vi "2283_mapaLIDAR.vi"(6 "Boolean Shift Register In":bool, 7 "Numeric Shift Register In":i32, 8 "X":dbl=350.0, 9 "# de Lecturas":i32=20) -> (1 "Boolean Shift Register Out":bool, 2 "Num Shift Register Out":i32)   [LabVIEW 2014]
uses:
  Mapa Global.vi
panel:
  out "Polar Plot":picture
  in  "Visible Section":u16(ring)=8
  in  "Grid Color":u32(colorbox)
  in  "Plot Color":u32(colorbox)=16715776
  out "Distance":dbl
  out "Mapa":cluster{dbl[], dbl[]}(graph)
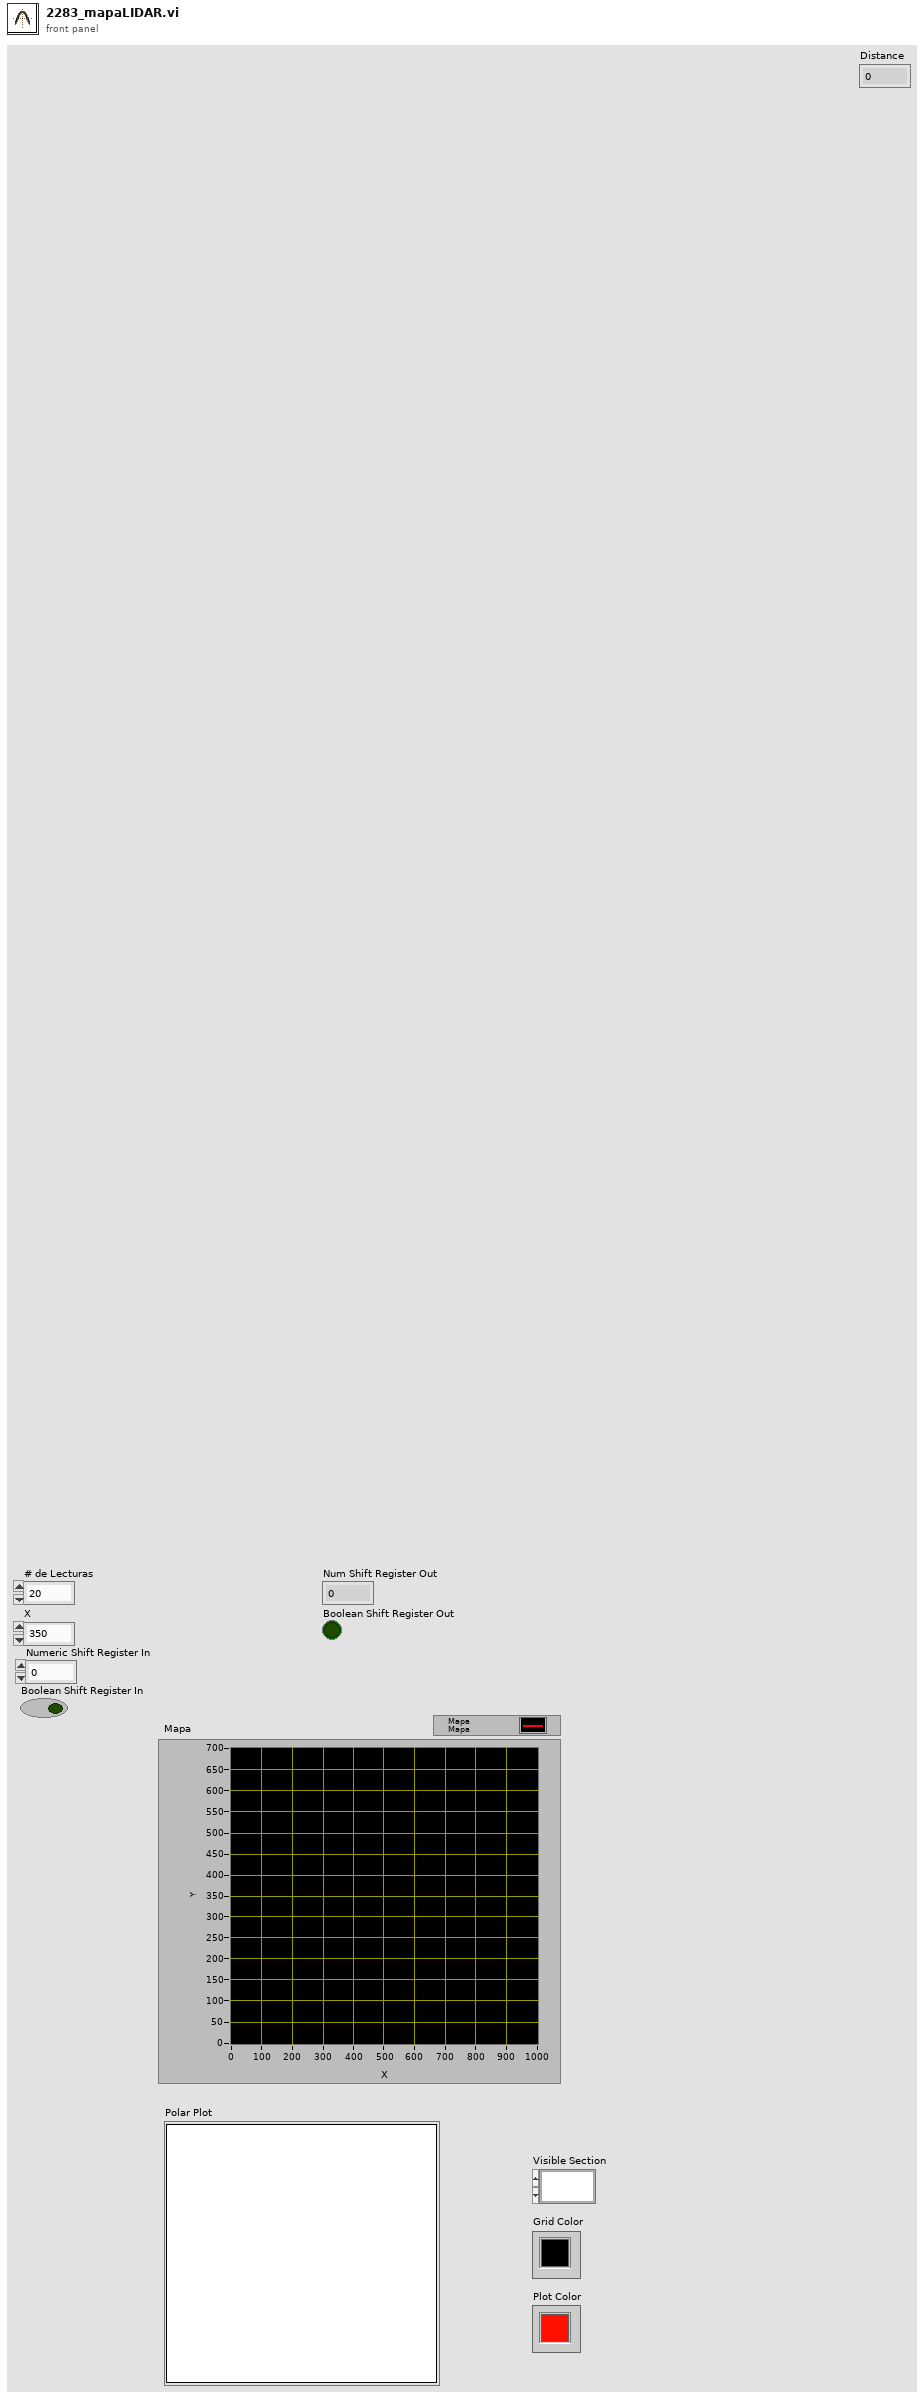
[diagram p1: front panel]
types:
  T1 = cluster{"maximum":dbl, "minimum":dbl, "clip to min":bool, "log?(F)":bool, "grid color":u32, "plot color":u32, "format and precision":cluster{"format":enum8{"Decimal", "Scientific", "Engineering", "Binary", "Octal", "Hex"}, "precision":u8}, "visible section":u16}
  T2 = typedef "WPI_I2CDevRef.ctl" = cluster{"DevStatus":errorcluster, "Controller":T3, "Device Address":u8, "Handle":i32, "I2C Bus":T4}
  T3 = typedef "FPGA_TypedefDigitalModule.ctl" = enum16{"Controller 1"}
  T4 = typedef "i2c_bus.ctl" = enum16{"I2C On-Board", "I2C MXP", "Invalid"}
  T5 = typedef "LVBoundsTypeDef.ctl" = cluster{"Width":u32, "Height":u32}
  T6 = typedef "WPI_ServoDeviceRef.ctl" = cluster{"DeviceStatus":errorcluster, "Controller":T3, "PWM Channel":T7, "DeadBand":T8}
  T7 = typedef "FPGA_DIOPWMChannel.ctl" = enum8{"PWM 0", "PWM 1", "PWM 2", "PWM 3", "PWM 4", "PWM 5", "PWM 6", "PWM 7", "PWM 8", "PWM 9", "PWM MXP 0", "PWM MXP 1", "PWM MXP 2", "PWM MXP 3", "PWM MXP 4", "PWM MXP 5", "PWM MXP 6", "PWM MXP 7", "PWM MXP 8", "PWM MXP 9", "Invalid"}
  T8 = typedef "WPI_PWMDeadband.ctl" = cluster{"Name":string, "maxPositivePwm":i32, "minPositivePwm":i32, "centerPwm":i32, "maxNegativePwm":i32, "minNegativePwm":i32, "angularRange":u16}
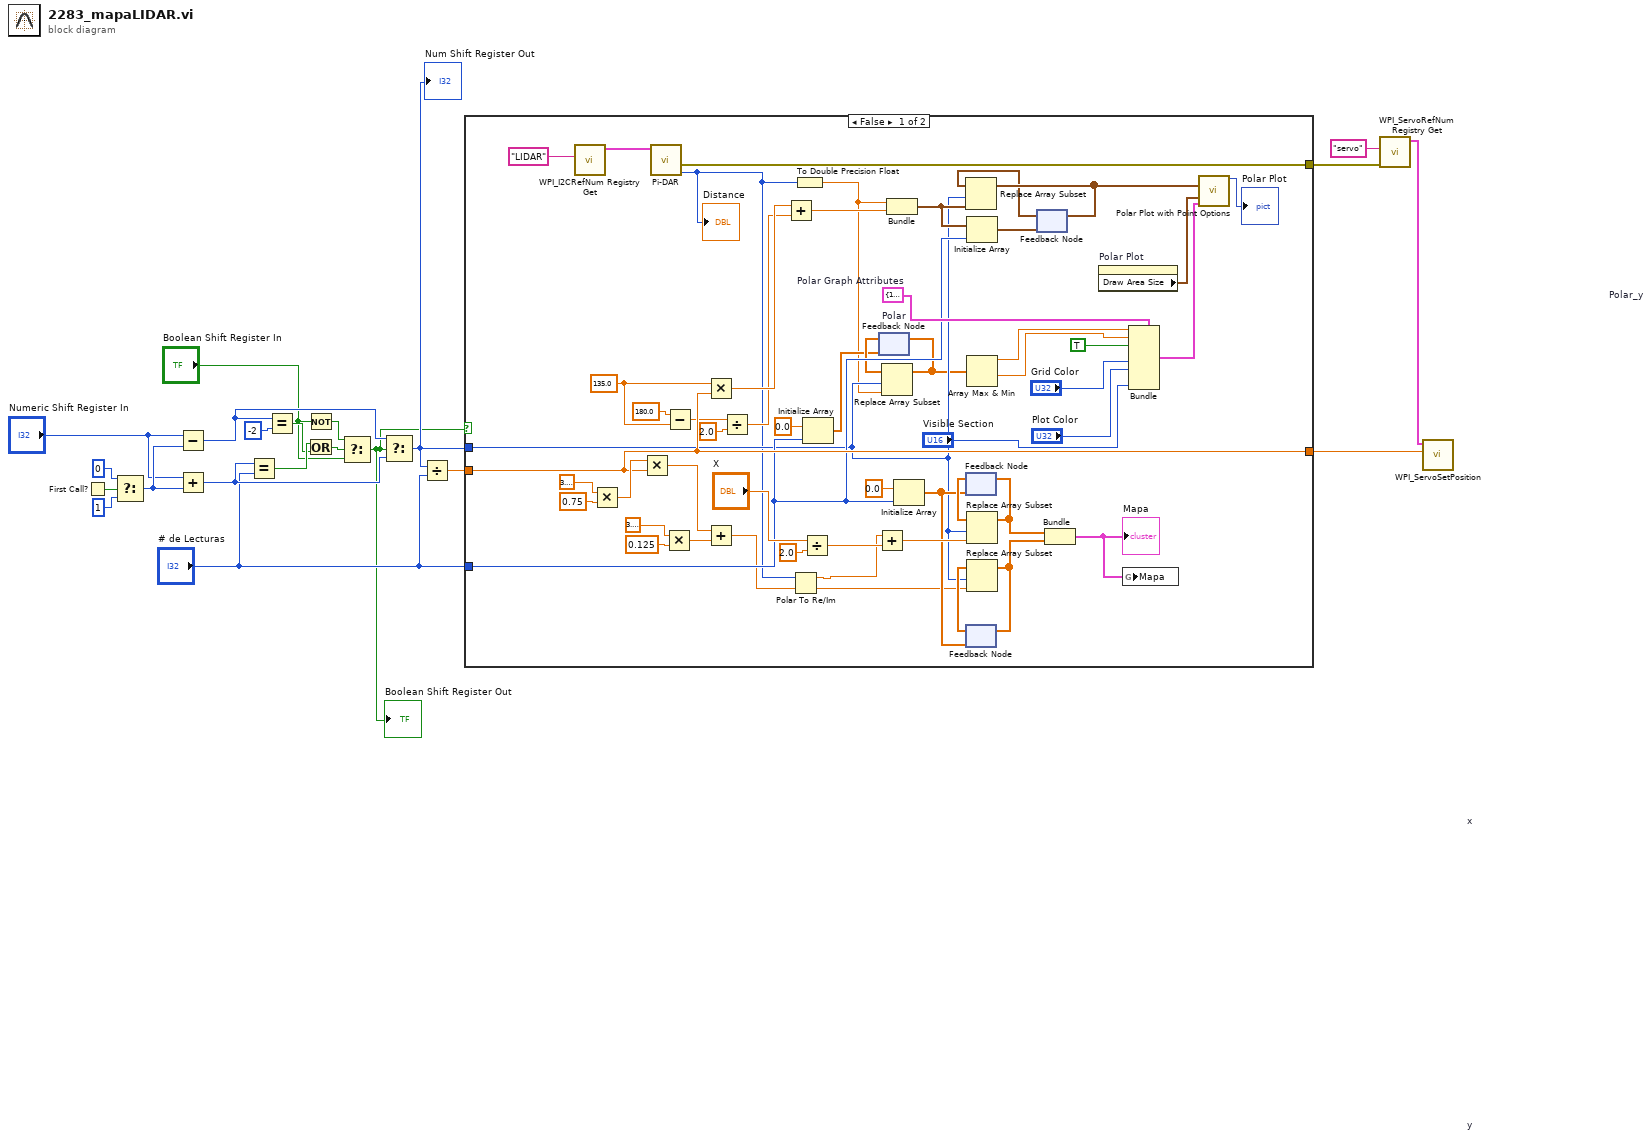
[diagram p0: block diagram]
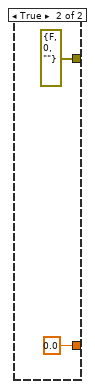
[diagram p2: hidden frame]
diagram:
  n1 = First Call?() -> (First Call?: T/F=w14:bool)
  n2 = Select(t=0, s=w14, f=1) -> (s? t:f=w11:i32)
  n3 = Subtract(x="Numeric Shift Register In", y=w11) -> (x-y=w16:i32)
  n4 = Add(x="Numeric Shift Register In", y=w11) -> (x+y=w15:i32)
  n5 = Equal?(x=w15, y="# de Lecturas") -> (x = y?=w19:bool)
  n6 = Equal?(x=w16, y=-2) -> (x = y?=w18:bool)
  n7 = Not(x="Boolean Shift Register In") -> (.not. x?=w20:bool)
  n8 = Or(x=w19, y=w18) -> (x .or. y?=w17:bool)
  n9 = Select(t=w20, s=w17, f="Boolean Shift Register In") -> (s? t:f=w1:bool)
  "Boolean Shift Register Out" <- w1
  n10 = Select(t=w16, s=w1, f=w15) -> (s? t:f=w9:i32)
  "Num Shift Register Out" <- w9
  n11 = Divide(x=w9, y="# de Lecturas") -> (x/y=w5:dbl)
  n12 = case shown="False" w1 {
    tunnel: w5 -> [w43 _]
    tunnel: "# de Lecturas" -> [w31 _]
    tunnel: w9 -> [w28 _]
    tunnel: [w56 errorcluster {"status"=FALSE, "code"=0, "source"=""} ("error out")] -> w6
    tunnel: [w43 0.0] -> w4
    frame False {
      w37 = 135.0
      w52 = T1 {"maximum"=1.0, "minimum"=0.0, "clip to min"=FALSE, "log?(F)"=FALSE, "grid color"=6710886, "plot color"=65280, "format and precision"={"format"=enum."Decimal", "precision"=1}, "visible section"=0}  # Polar Graph Attributes
      n13 = call <vilib>:"WPI_I2CRefNum Registry Get.vi"("refnum name"="LIDAR") -> ("I2CDevRef"=w61:T2)  [unwired: 9 in, 1 out]
      n14 = Multiply(x=3.141592653589793, y=0.75 ("x")) -> (x*y=w67:dbl)
      n15 = Multiply(x=w67, y=w43) -> (x*y=w75:dbl)
      n16 = call "Pi-DAR.vi"("I2CDevRef"=w61) -> ("Distance Output"=w25:i32, "error out"=w56:errorcluster)  [unwired: 9 in]
      "Distance" <- w25
      n17 = Multiply(x=3.141592653589793, y=0.125 ("x")) -> (x*y=w66:dbl)
      n18 = Subtract(x=180.0, y=w37) -> (x-y=w41:dbl)
      n19 = Multiply(x=w37, y=w43) -> (x*y=w44:dbl)
      n20 = Add(x=w75, y=w66) -> (x+y=w24:dbl)
      n21 = Divide(x=w41, y=2.0) -> (x/y=w40:dbl)
      n22 = Add(x=w44, y=w40) -> (x+y=w42:dbl)
      n23 = Polar To Re/Im(2:w24, 3:w25) -> (0:w22:dbl, 1:w23:dbl)
      n24 = To Double Precision Float(number=w25) -> (double precision float=w27:dbl)
      n25 = Divide(x="X", y=2.0) -> (x/y=w59:dbl)
      n26 = Initialize Array(0.0 ("element"), w31) -> (w29:dbl[])
      n27 = Add(x=w23, y=w59) -> (x+y=w64:dbl)
      n28 = feedback #1 "Polar"(w29) -> (w30:dbl[])
      n29 = Replace Array Subset(array=w30, new element=w27, index=w28) -> (w26:dbl[])
      n30 = feedback-in #1(w26) -> ()
      n31 = Bundle(w27, w42) -> (w47:cluster{dbl, dbl})  [unwired: 1 in]
      n32 = Initialize Array(0.0 ("element"), w31) -> (w55:dbl[])
      n33 = feedback #2 "x"(w55) -> (w65:dbl[])
      n34 = feedback #3 "y"(w55) -> (w72:dbl[])
      n35 = Initialize Array(w47, w31) -> (w54:cluster{dbl, dbl}[])
      n36 = Array Max & Min(array=w26) -> (max value=w34:dbl, min value=w33:dbl)  [unwired: 2 out]
      n37 = Replace Array Subset(array=w65, new element=w64, index=w28) -> (w63:dbl[])
      n38 = feedback-in #2(w63) -> ()
      n39 = Replace Array Subset(array=w72, new element=w22, index=w28) -> (w71:dbl[])
      n40 = feedback-in #3(w71) -> ()
      n41 = feedback #4 "Polar_y"(w54) -> (w35:cluster{dbl, dbl}[])
      n42 = Replace Array Subset(array=w35, new element=w47, index=w28) -> (w53:cluster{dbl, dbl}[])
      n43 = feedback-in #4(w53) -> ()
      n44 = Bundle(w63, w71) -> (w60:cluster{dbl[], dbl[]})  [unwired: 1 in]
      "Mapa" <- w60
      n45 = property on="Polar Plot" class="Pict"() -> ("Draw Area Size"=w46:T5)  [unwired: 2 in, 2 out]
      n46 = global write "Mapa Global.vi" "Mapa"(w60) -> ()
      n47 = Bundle(cluster=w52, "maximum"=w34, "minimum"=w33, "clip to min"=TRUE, "grid color"="Grid Color", "plot color"="Plot Color", "visible section"="Visible Section") -> (w48:T1)  [unwired: 2 in]
      n48 = call <vilib>:"Polar Plot with Point Options.vi"("data array [mag, phase (deg)]"=w53, "dimensions (w,h)"=w46, "polar attributes"=w48) -> ("new picture"=→"Polar Plot":picture)  [unwired: 12 in]
    }
    frame True {
    }
  }
  n49 = call <vilib>:"WPI_ServoRefNum Registry Get.vi"("error in (no error)"=w6, "refnum name"="servo") -> ("ServoDeviceRef"=w7:T6)  [unwired: 8 in, 1 out]
  n50 = call <vilib>:"WPI_ServoSetPosition.vi"("Position"=w4, "ServoDeviceRef"=w7) -> ()  [unwired: 8 in, 2 out]
